vi "GetPTInfo.vi"(2 "错误输出":errorcluster, 3 "Page引用句柄":refnum<vi>) -> (0 "error out":errorcluster, 1 "PT values":dbl[](array[numeric]))   [LabVIEW 2017]
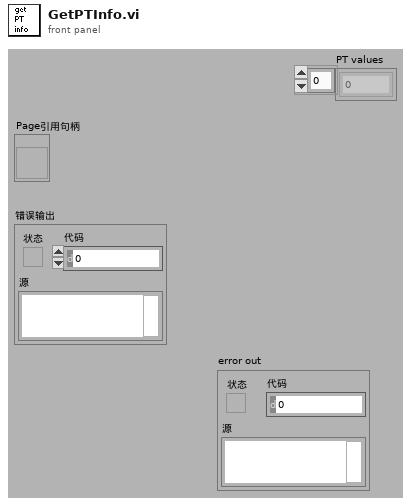
[diagram p1: front panel]
types:
  T1 = cluster{"类型":dbl, "类型 2":dbl, "类型 3":dbl, "类型 4":dbl}
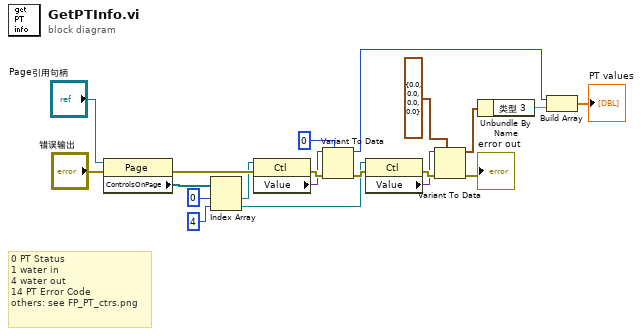
[diagram p0: block diagram]
diagram:
  # "0 PT Status\n1 water in\n4 water out \n14 PT Error Code\nothers: see FP_PT_ctrs.png"
  n1 = property class="Page"(reference="Page引用句柄", error in="错误输出") -> (error out=w19:errorcluster, "ControlsOnPage"=w8:refnum<vi>[])  [unwired: 1 out]
  n2 = Index Array(array=w8, index #1=0 ("索引"), index #2=4 ("索引")) -> (element #1=w10:refnum<vi>, element #2=w4:refnum<vi>)
  n3 = property class="Ctl"(reference=w10, error in=w19) -> (error out=w17:errorcluster, "Value"=w11:variant)  [unwired: 1 out]
  n4 = Variant To Data(error in=w17, type=0 ("类型"), Variant=w11) -> (data=w2:i32, error out=w6:errorcluster)
  n5 = property class="Ctl"(reference=w4, error in=w6) -> (error out=w18:errorcluster, "Value"=w13:variant)  [unwired: 1 out]
  n6 = Variant To Data(error in=w18, type=T1 {"类型"=0.0, "类型 2"=0.0, "类型 3"=0.0, "类型 4"=0.0}, Variant=w13) -> (data=w14:T1, error out=→"error out":errorcluster)
  n7 = Unbundle By Name(w14) -> ("类型 3"=w3:dbl)
  n8 = Build Array(w2, w3) -> (→"PT values":dbl[])
